vi "Fieldscan measurement.vi"(8 "error in (no error)":errorcluster, 11 "Cmd string":string) -> (0 "error out":errorcluster)   [LabVIEW 2019]
doc: "Nicolas Weiss - EPFL - IPHYS 2019\n----\nThis VI performs data acquisition while the field is ramping from Bstart to Bend."
uses:
  Controls/Save data file action.ctl
  Controls/Plot data action.ctl
  Controls/Data to save cluster.ctl
  _Global variables 1.vi
panel:
  out "Data acquisition interval (s)":dbl
  out "Temperature (K)":dbl
  out "Field (T)":dbl
  out "Status":string
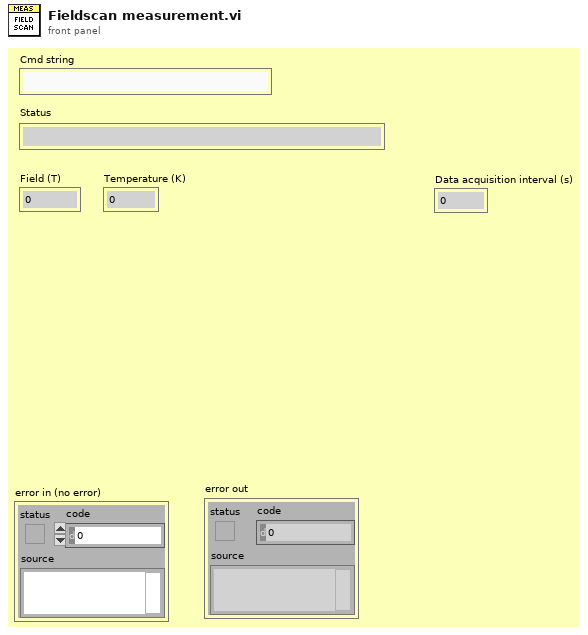
[diagram p1: front panel]
types:
  T1 = typedef "Plot data action.ctl" = enum16{"init graph", "Append data"}
  T2 = typedef "Save data file action.ctl" = enum16{"Create & init file", "Append data", "Close file"}
  T3 = typedef "Data to save cluster.ctl" = cluster{"Magnetic field 1 T)":dbl, "Magnetic field 2 (T)":dbl, "Temperature 1 (K)":dbl, "Temperature 2 (K)":dbl, "Lock-in amplifier 1 (uV)":dbl, "Lock-in amplifier 2 (uV)":dbl, "ZVL power":dbl, "ZVL attenuation":dbl, "ZVL data array 1 {Freq}{Real}{Imag} [N seg at const field]":string[], "ZVL data array 2 {Freq}{Real}{Imag} [N seg at const field]":string[]}
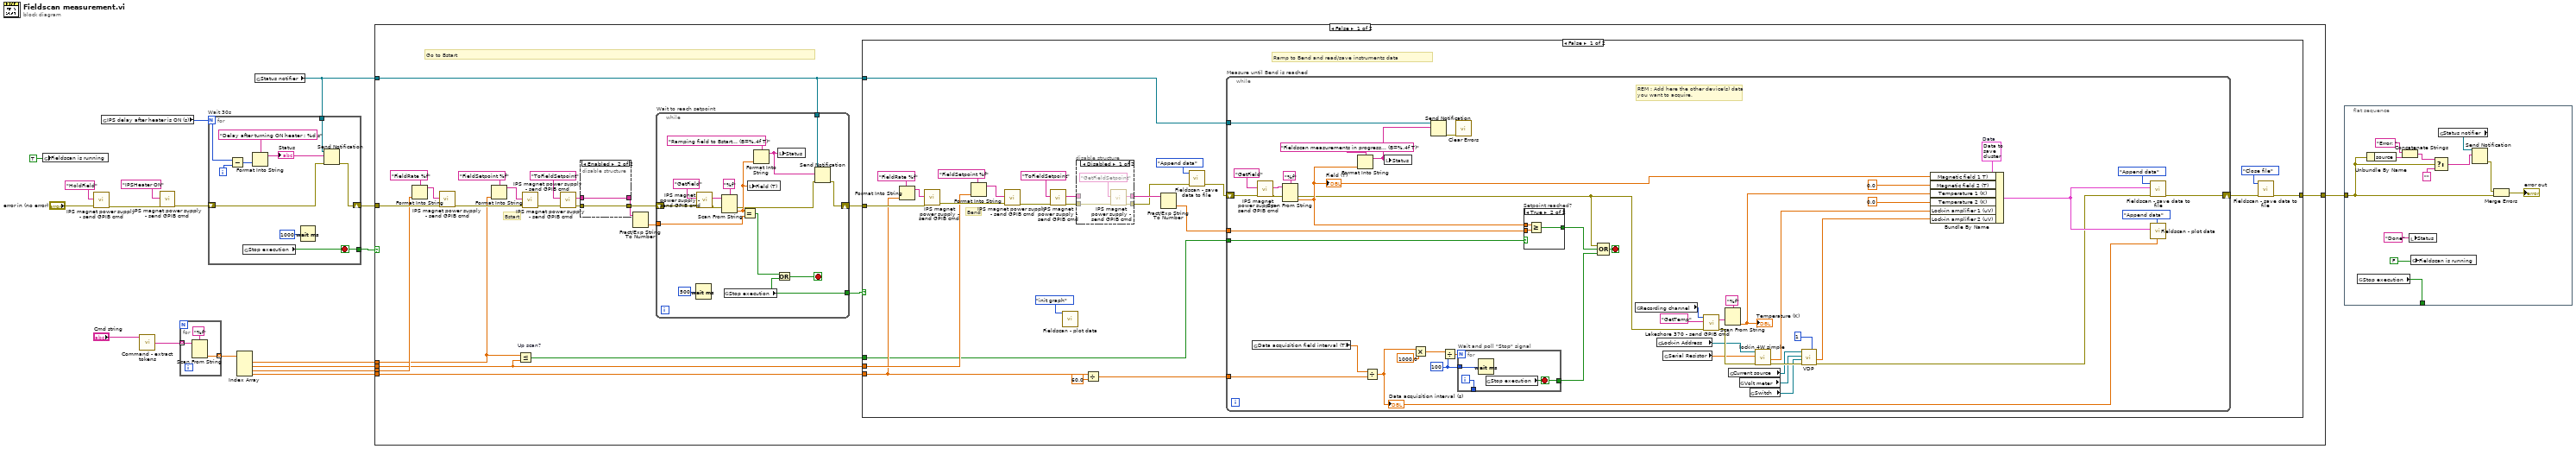
[diagram p0: block diagram]
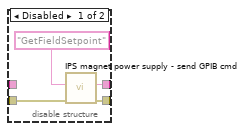
[diagram p2: hidden frame]
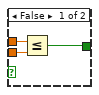
[diagram p4: hidden frame]
diagram:
  n1 = global write "_Global variables 1.vi" "Fieldscan is running"(TRUE ("Scan is running")) -> ()
  n2 = call "IPS magnet power supply - send GPIB cmd.vi"("error in (no error)"="error in (no error)", "Cmd string"="HoldField") -> ("error out"=w15:errorcluster)  [unwired: 8 in, 1 out]
  n3 = global read "_Global variables 1.vi" "IPS delay after heater is ON (s)"() -> (w9:i32)
  n4 = call "Command - extract tokens.vi"("Cmd string"="Cmd string") -> ("Arguments"=w7:string[])  [unwired: 2 in, 2 out]
  n5 = call "IPS magnet power supply - send GPIB cmd.vi"("error in (no error)"=w15, "Cmd string"="IPSHeater ON") -> ("error out"=w14:errorcluster)  [unwired: 8 in, 1 out]
  n6 = for {
    tunnel: w7 -> [w20] mode=indexing
    tunnel: [w19] -> w6 mode=indexing
    n7 = Scan From String(format string="%f", input string=w20) -> (output 1=w19:dbl)  [unwired: 3 in, 3 out]
  }
  n8 = Index Array(array=w6) -> (element #1=w5:dbl, element #2=w3:dbl, element #3=w4:dbl, element #4=w2:dbl)  [unwired: 4 in]
  n9 = global read "_Global variables 1.vi" "Status notifier"() -> (w1:refnum<notifier>)
  n10 = for "Wait 30s" {
    N: w9 -> [w26]
    tunnel: [w30] -> w11
    tunnel: w1 -> [w25]
    shift-right: [w22] -> w13
    shift-left: w14 -> [w23]
    i -> [w28]
    stop <- w30 stop-if-true
    n11 = Subtract(x=w26, y=w28) -> (x-y=w27:i32)
    n12 = global read "_Global variables 1.vi" "Stop execution"() -> (w30:bool)
    n13 = Format Into String(format string="Delay after turning ON heater : %d s" ("Status"), w27) -> (resulting string=w24:string)  [unwired: 2 in, 1 out]
    "Status" <- w24
    n14 = Wait (ms)(milliseconds to wait=u32 1000) -> ()  [unwired: 1 out]
    n15 = Send Notification(notification=w24, notifier=w25, error in (no error)=w23) -> (error out=w22:errorcluster)  [unwired: 1 out]
  }
  n16 = case shown="False" w11 {
    tunnel: w13 -> [w53 w163]
    tunnel: [w40 w163] -> w12
    tunnel: w5 -> [w34 _]
    tunnel: w4 -> [w38 _]
    tunnel: w3 -> [w33 _]
    tunnel: w2 -> [w37 _]
    tunnel: w1 -> [w36 _]
    frame False {
      # "Bstart"
      # "Go to Bstart"
      n17 = Format Into String(format string="FieldRate %f" ("Cmd string"), w38) -> (resulting string=w51:string)  [unwired: 2 in, 1 out]
      n18 = call "IPS magnet power supply - send GPIB cmd.vi"("error in (no error)"=w53, "Cmd string"=w51) -> ("error out"=w48:errorcluster)  [unwired: 8 in, 1 out]
      n19 = Format Into String(format string="FieldSetpoint %f" ("Cmd string"), w34) -> (resulting string=w49:string)  [unwired: 2 in, 1 out]
      n20 = Less Or Equal? "Up scan?"(x=w34, y=w33) -> (x <= y?=w32:bool)
      n21 = call "IPS magnet power supply - send GPIB cmd.vi"("error in (no error)"=w48, "Cmd string"=w49) -> ("error out"=w47:errorcluster)  [unwired: 8 in, 1 out]
      n22 = call "IPS magnet power supply - send GPIB cmd.vi"("error in (no error)"=w47, "Cmd string"="ToFieldSetpoint") -> ("error out"=w45:errorcluster, "Response"=w35:string)  [unwired: 8 in]
      n23 = disable-structure shown="Enabled" {
        disable-tunnel: w45 -> [w57 w59]
        disable-tunnel: [w56 w59] -> w44
        disable-tunnel: [w54 w58] -> w43
        disable-tunnel: w35 -> [_ w58]
        frame Disabled {
          n24 = call "IPS magnet power supply - send GPIB cmd.vi"("error in (no error)"=w57, "Cmd string"="GetFieldSetpoint") -> ("error out"=w56:errorcluster, "Response"=w54:string)  [unwired: 8 in]
        }
        frame Enabled {
        }
      }
      n25 = Fract/Exp String To Number(string=w43) -> (number=w42:dbl)  [unwired: 3 in, 1 out]
      n26 = while "Wait to reach setpoint" {
        shift-right: [w149] -> w41
        shift-left: w44 -> [w161]
        tunnel: w42 -> [w154]
        tunnel: [w153] -> w39
        tunnel: w36 -> [w150]
        stop <- w156 stop-if-true
        n27 = Wait (ms)(milliseconds to wait=u32 500) -> ()  [unwired: 1 out]
        n28 = call "IPS magnet power supply - send GPIB cmd.vi"("error in (no error)"=w161, "Cmd string"="GetField") -> ("error out"=w148:errorcluster, "Response"=w159:string)  [unwired: 8 in]
        n29 = Scan From String(format string="%f", input string=w159, error in=w148) -> (error out=w147:errorcluster, output 1=w152:dbl)  [unwired: 2 in, 2 out]
        n30 = global read "_Global variables 1.vi" "Stop execution"() -> (w153:bool)
        n31 = Equal?(x=w152, y=w154) -> (x = y?=w157:bool)
        n32 = local write "Field (T)"(w152) -> ()
        n33 = Format Into String(format string="Ramping field to Bstart... (B=%.4f T)" ("Status"), w152) -> (resulting string=w151:string)  [unwired: 2 in, 1 out]
        n34 = Or(x=w157, y=w153) -> (x .or. y?=w156:bool)
        n35 = local write "Status"(w151) -> ()
        n36 = Send Notification(notification=w151, notifier=w150, error in (no error)=w147) -> (error out=w149:errorcluster)  [unwired: 1 out]
      }
      n37 = case shown="False" w39 {
        tunnel: w41 -> [w75 w146]
        tunnel: [w70 w146] -> w40
        tunnel: w33 -> [w68 _]
        tunnel: w37 -> [w65 _]
        tunnel: w36 -> [w67 _]
        tunnel: w32 -> [w60 _]
        frame False {
          # "Bend"
          # "Ramp to Bend and read/save instruments data"
          n38 = Format Into String(format string="FieldRate %f" ("Cmd string"), w65) -> (resulting string=w84:string)  [unwired: 2 in, 1 out]
          n39 = call "IPS magnet power supply - send GPIB cmd.vi"("error in (no error)"=w75, "Cmd string"=w84) -> ("error out"=w82:errorcluster)  [unwired: 8 in, 1 out]
          n40 = Format Into String(format string="FieldSetpoint %f" ("Cmd string"), w68) -> (resulting string=w83:string)  [unwired: 2 in, 1 out]
          n41 = call "IPS magnet power supply - send GPIB cmd.vi"("error in (no error)"=w82, "Cmd string"=w83) -> ("error out"=w81:errorcluster)  [unwired: 8 in, 1 out]
          n42 = call "IPS magnet power supply - send GPIB cmd.vi"("error in (no error)"=w81, "Cmd string"="ToFieldSetpoint") -> ("error out"=w80:errorcluster, "Response"=w66:string)  [unwired: 8 in]
          n43 = call "Fieldscan - plot data.vi"("Action"=Plot_data_action."init graph") -> ()  [unwired: 10 in, 1 out]
          n44 = disable-structure shown="Disabled" {
            disable-tunnel: w80 -> [w88 w90]
            disable-tunnel: [w87 w89] -> w79
            disable-tunnel: [w85 w90] -> w62
            disable-tunnel: w66 -> [_ w89]
            frame Disabled {
              n45 = call "IPS magnet power supply - send GPIB cmd.vi"("error in (no error)"=w88, "Cmd string"="GetFieldSetpoint") -> ("error out"=w85:errorcluster, "Response"=w87:string)  [unwired: 8 in]
            }
            frame Enabled {
            }
          }
          n46 = Divide(x=w65, y=60.0) -> (x/y=w63:dbl)
          n47 = Fract/Exp String To Number(string=w79) -> (number=w74:dbl)  [unwired: 3 in, 1 out]
          n48 = call "Fieldscan - save data to file.vi"("error in (no error)"=w62, "Action"=Save_data_file_action."Append data") -> ("error out"=w72:errorcluster)  [unwired: 8 in, 1 out]
          n49 = while "Measure until Bend is reached" {
            shift-right: [w131] -> w71
            shift-left: w72 -> [w136]
            tunnel: w74 -> [w107]
            tunnel: w67 -> [w125]
            tunnel: w63 -> [w118]
            tunnel: w60 -> [w108]
            stop <- w132 stop-if-true
            w104 = u32 100 ("milliseconds to wait")
            w116 = T3 {"Magnetic field 1 T)"=0.0, "Magnetic field 2 (T)"=0.0, "Temperature 1 (K)"=0.0, "Temperature 2 (K)"=0.0, "Lock-in amplifier 1 (uV)"=0.0, "Lock-in amplifier 2 (uV)"=0.0, "ZVL power"=0.0, "ZVL attenuation"=0.0, "ZVL data array 1 {Freq}{Real}{Imag} [N seg at const field]"=[], "ZVL data array 2 {Freq}{Real}{Imag} [N seg at const field]"=[]}  # Data
            # "REM : Add here the other device(s) data\nyou want to acquire."
            n50 = global read "_Global variables 1.vi" "Data acquisition field interval (T)"() -> (w117:dbl)
            n51 = call "IPS magnet power supply - send GPIB cmd.vi"("error in (no error)"=w136, "Cmd string"="GetField") -> ("error out"=w123:errorcluster, "Response"=w134:string)  [unwired: 8 in]
            n52 = Scan From String(format string="%f", input string=w134, error in=w123) -> (error out=w92:errorcluster, output 1=w106:dbl)  [unwired: 2 in, 2 out]
            "Field (T)" <- w106
            n53 = Format Into String(format string="Fieldscan measurements in progress... (B=%.4f T)" ("Status"), w106) -> (resulting string=w124:string)  [unwired: 2 in, 1 out]
            n54 = Divide(x=w117, y=w118) -> (x/y=w101:dbl)
            "Data acquisition interval (s)" <- w101
            n55 = local write "Status"(w124) -> ()
            n56 = Multiply(x=w101, y=1000.0) -> (x*y=w102:dbl)
            n57 = Send Notification(notification=w124, notifier=w125) -> (error out=w114:errorcluster)  [unwired: 1 in, 1 out]
            n58 = Divide(x=w102, y=w104) -> (x/y=w103:dbl)
            n59 = call <vilib>:"Clear Errors.vi"("error in (no error)"=w114) -> ()  [unwired: 5 in, 2 out]
            n60 = for "Wait and poll \"Stop\" signal" {
              N: w103 -> [_]
              tunnel: [w139] -> _
              tunnel: w104 -> [w138]
              tunnel: [w137] -> w100
              i -> [w139]
              stop <- w137 stop-if-true
              n61 = Wait (ms)(milliseconds to wait=w138) -> ()  [unwired: 1 out]
              n62 = global read "_Global variables 1.vi" "Stop execution"() -> (w137:bool)
            }
            n63 = case "Setpoint reached?" shown="True" w108 {
              tunnel: w107 -> [w141 w144]
              tunnel: w106 -> [w142 w145]
              tunnel: [w140 w143] -> w105
              frame False {
                n64 = Less Or Equal?(x=w142, y=w141) -> (x <= y?=w140:bool)
              }
              frame True {
                n65 = Greater Or Equal?(x=w145, y=w144) -> (x >= y?=w143:bool)
              }
            }
            n66 = Compound Arithmetic op=OR(w92, w105, w100) -> (w132:bool)
            n67 = global read "_Global variables 1.vi" "Recording channel"() -> (w91:enum16{"Sample stage", "Mixing chamber"})
            n68 = global read "_Global variables 1.vi" "Lock-in Address"() -> (w121:refnum<visa-resource-name>)
            n69 = global read "_Global variables 1.vi" "Serial Resistor"() -> (w120:dbl)
            n70 = call "Lakeshore 370 - send GPIB cmd.vi"("error in (no error)"=w92, "Cmd string"="GetTemp", "Enum"=w91) -> ("error out"=w122:errorcluster, "Response"=w128:string)  [unwired: 7 in]
            n71 = Scan From String(format string="%f", input string=w128) -> (output 1=w111:dbl)  [unwired: 3 in, 3 out]
            "Temperature (K)" <- w111
            n72 = global read "_Global variables 1.vi" "Current source"() -> (w93:refnum<visa-resource-name>)
            n73 = global read "_Global variables 1.vi" "Volt meter"() -> (w95:refnum<visa-resource-name>)
            n74 = global read "_Global variables 1.vi" "Switch"() -> (w94:refnum<visa-resource-name>)
            n75 = call "lockin 4W simple.vi"("error in (no error)"=w122, "serial resistor"=w120, "VISA lockin"=w121) -> ("error out"=w99:errorcluster, "resistance"=w110:dbl)  [unwired: 6 in, 1 out]
            n76 = call "VDP.vi"("Settling time"=u32 1, "error in (no error)"=w99, "VISA scanner"=w94, "VISA nanoVM"=w95, "VISA current"=w93) -> ("error out"=w98:errorcluster, "sheet resistance"=w97:dbl)  [unwired: 5 in]
            n77 = Bundle By Name(cluster=w116, "Magnetic field 1 T)"=w106, "Magnetic field 2 (T)"=0.0, "Temperature 1 (K)"=w111, "Temperature 2 (K)"=0.0, "Lock-in amplifier 1 (uV)"=w110, "Lock-in amplifier 2 (uV)"=w97) -> (w109:T3)
            n78 = call "Fieldscan - save data to file.vi"("error in (no error)"=w98, "Data"=w109, "Action"=Save_data_file_action."Append data") -> ("error out"=w131:errorcluster)  [unwired: 7 in, 1 out]
            n79 = call "Fieldscan - plot data.vi"("Data acquisition interval (s)"=w101, "Data"=w109, "Action"=Plot_data_action."Append data") -> ()  [unwired: 8 in, 1 out]
          }
          n80 = call "Fieldscan - save data to file.vi"("error in (no error)"=w71, "Action"=Save_data_file_action."Close file") -> ("error out"=w70:errorcluster)  [unwired: 8 in, 1 out]
        }
        frame True {
        }
      }
    }
    frame True {
    }
  }
  n81 = flat-sequence {
    tunnel: w12 -> [w169]
    tunnel: [w164] -> _
    frame #0 {
      n82 = global read "_Global variables 1.vi" "Stop execution"() -> (w164:bool)
      n83 = Unbundle By Name(w169) -> ("source"=w168:string)
      n84 = Concatenate Strings("Error: " ("Status"), w168) -> (w166:string)
      n85 = local write "Status"("Done" ("Status")) -> ()
      n86 = global write "_Global variables 1.vi" "Fieldscan is running"(FALSE ("Scan is running")) -> ()
      n87 = Select(t=w166, s=w169, f="" ("Status")) -> (s? t:f=w165:string)
      n88 = global read "_Global variables 1.vi" "Status notifier"() -> (w174:refnum<notifier>)
      n89 = Send Notification(notification=w165, notifier=w174) -> (error out=w171:errorcluster)  [unwired: 1 in, 1 out]
      n90 = Merge Errors(w171, w169) -> (→"error out":errorcluster)
    }
  }
